vi "SCMP CoMP-S Mechanism - focus.vi"(8 "error in (no error)":errorcluster, 9 "Auto Motors":bool, 10 "Old Focus":T1=70.0 min=70.0 max=152.0 format="%.2f", 11 "Desired Focus":T1 min=70.0 max=152.0 format="%.2f") -> (0 "error out":errorcluster, 3 "Focus out":dbl)   [LabVIEW 2014]
uses:
  Controls/focus.ctl
panel:
  # "Moving Focus\n  wait please"
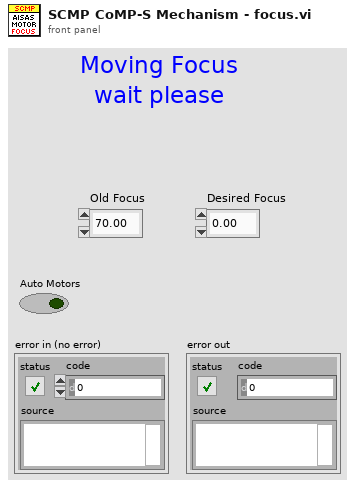
[diagram p1: front panel]
types:
  T1 = typedef "focus.ctl" = dbl
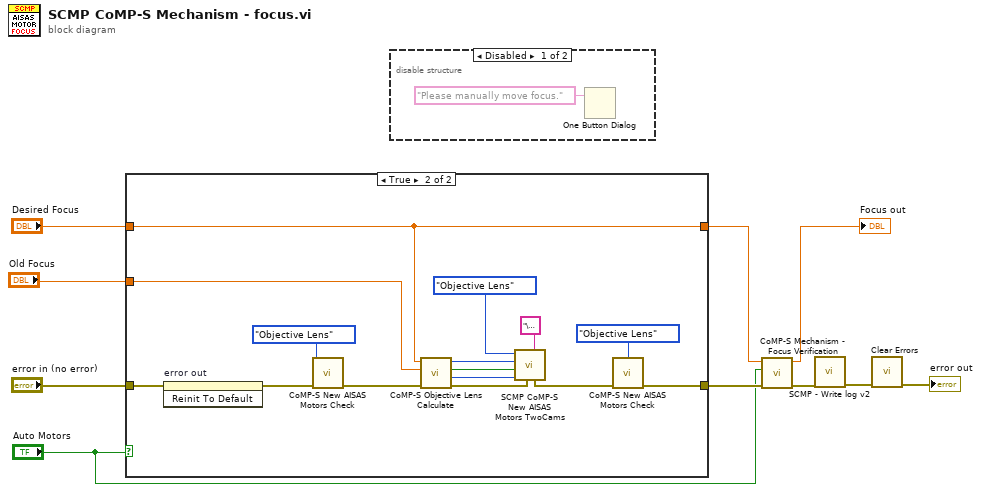
[diagram p0: block diagram]
diagram:
  n1 = case shown="True" "Auto Motors" {
    tunnel: "error in (no error)" -> [w12 w27]
    tunnel: "Old Focus" -> [_ w26]
    tunnel: [w12 w14] -> w9
    tunnel: "Desired Focus" -> [w11 w13]
    tunnel: [w11 w13] -> w2
    frame False {
    }
    frame True {
      n2 = invoke on="error out" class="Clust (strict)" method="Reinit To Default"(error in=w27) -> (error out=w15:errorcluster)  [unwired: 2 in, 2 out]
      n3 = call "CoMP-S New AISAS Motors Check.vi"("error in (no error)"=w15, "Motor selection"=enum32{"Rotation", "Difuser ", "Objective Lens"}."Objective Lens") -> ("error out"=w20:errorcluster)  [unwired: 9 in]
      n4 = call "CoMP-S Objective Lens Calculate.vi"("error in (no error)"=w20, "old Focus"=w26, "new Focus"=w13) -> ("error out"=w19:errorcluster, "Velocity"=w18:i32, "Motor Direction"=w17:bool, "Steps"=w16:i32)  [unwired: 4 in]
      n5 = call "SCMP CoMP-S New AISAS Motors TwoCams.vi"("Motion Code"="\u0002", "error in (no error)"=w19, "steps/sec"=w18, "motor rotation"=w17, "Steps"=w16, "Motor selection"=enum32{"Rotation", "Difuser ", "Objective Lens"}."Objective Lens") -> ("error out"=w23:errorcluster)  [unwired: 2 in, 3 out]
      n6 = call "CoMP-S New AISAS Motors Check.vi"("error in (no error)"=w23, "Motor selection"=enum32{"Rotation", "Difuser ", "Objective Lens"}."Objective Lens") -> ("error out"=w14:errorcluster)  [unwired: 9 in]
    }
  }
  n7 = disable-structure shown="Disabled" {
    frame Disabled {
      n8 = One Button Dialog(message="Please manually move focus.") -> ()  [unwired: 1 in, 1 out]
    }
    frame Enabled {
    }
  }
  n9 = call "CoMP-S Mechanism - Focus Verification.vi"("error in (no error)"=w9, "Motors"="Auto Motors", "Focus"=w2) -> ("error out"=w7:errorcluster, "Focus out"=→"Focus out":dbl)  [unwired: 7 in]
  n10 = call "SCMP - Write log v2.vi"("Error to log"=w7) -> ("error out"=w8:errorcluster)  [unwired: 8 in, 2 out]
  n11 = call <vilib>:"Clear Errors.vi"("error in (no error)"=w8) -> ("error out"=→"error out":errorcluster)  [unwired: 5 in, 1 out]
